vi "parametryKomor.vi"(3 "Akcja":T1, 4 "Wybór komory":T6, 5 "Wejœcie":T2={"Pinout"={"LEWO"=7, "PRAWO"=11, "GÓRA"=35, "Dӣ"=36, "CZUJNIK"=12}, "Parametry ruchu poziomego"={"Faza ruchu poziomego"=enum."Ruch", "Nr pozycji poziomej"=0, "Kolor czujnika"=FALSE, "Lista punków w poziomie"=[]}, "Parametry ruchy pionowego"={"Faza ruchu"=enum."Ruch", "Lista punktów w pionie"=[]}}) -> (2 "Wyjscie":T2={"Pinout"={"LEWO"=7, "PRAWO"=11, "GÓRA"=35, "Dӣ"=36, "CZUJNIK"=12}, "Parametry ruchu poziomego"={"Faza ruchu poziomego"=enum."Ruch", "Nr pozycji poziomej"=0, "Kolor czujnika"=FALSE, "Lista punków w poziomie"=[]}, "Parametry ruchy pionowego"={"Faza ruchu"=enum."Ruch", "Lista punktów w pionie"=[]}})   [LabVIEW 2014]
uses:
  parametryKomorVIs/WyborKomory.ctl
  parametryKomorVIs/Parametry_ramienia.ctl
  poziomyVIs/ParametryRuchuPoziomego.ctl
  Faza_ruchu.ctl
  pionowyVIs/ParametryRuchyPionowego.ctl
  AkcjaGFV.ctl
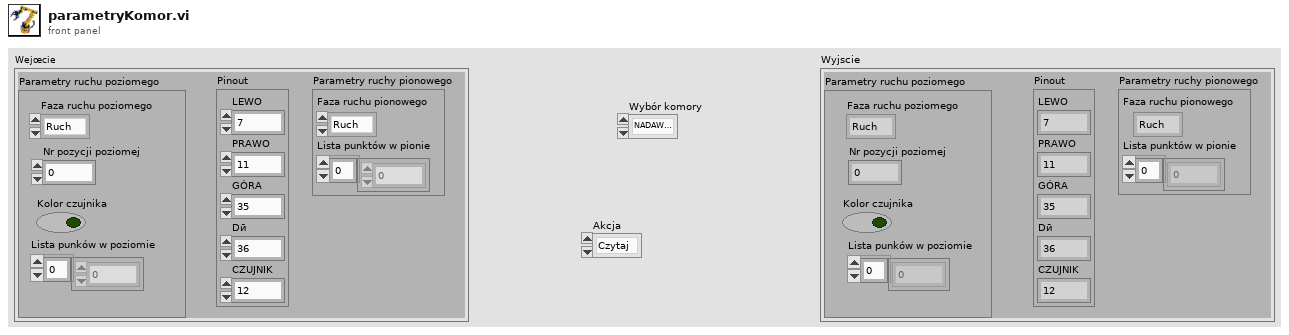
[diagram p1: front panel]
types:
  T1 = typedef "AkcjaGFV.ctl" = enum16{"Czytaj", "Zapisz", "Reset"}
  T2 = typedef "Parametry_ramienia.ctl" = cluster{"Pinout":cluster{"LEWO":u8, "PRAWO":u8, "GÓRA":u8, "Dӣ":u8, "CZUJNIK":u8}, "Parametry ruchu poziomego":T3, "Parametry ruchy pionowego":T5}
  T3 = typedef "ParametryRuchuPoziomego.ctl" = cluster{"Faza ruchu poziomego":T4, "Nr pozycji poziomej":i32, "Kolor czujnika":bool, "Lista punków w poziomie":i32[]}
  T4 = typedef "Faza_ruchu.ctl" = enum16{"Ruch", "Poczekaj", "Pomiar"}
  T5 = typedef "ParametryRuchyPionowego.ctl" = cluster{"Faza ruchu":T4, "Lista punktów w pionie":i32[]}
  T6 = typedef "WyborKomory.ctl" = enum16{"NADAWCZA", "ODBIORCZA"}
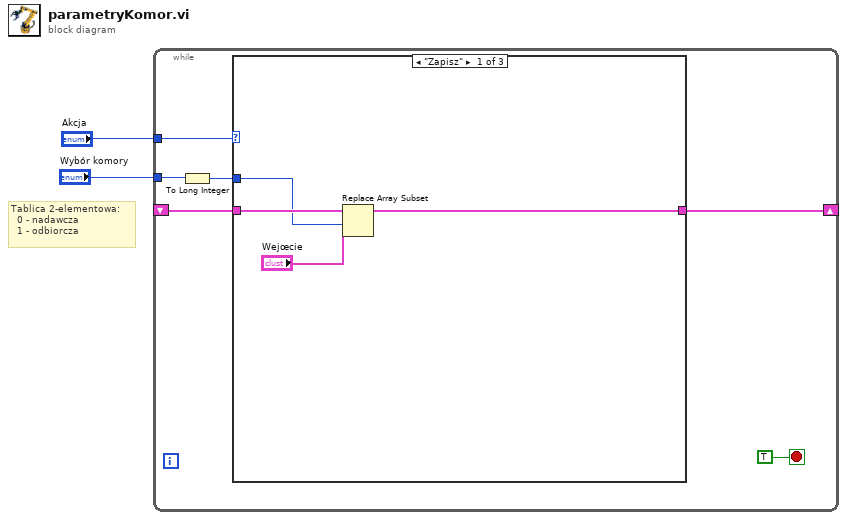
[diagram p0: block diagram]
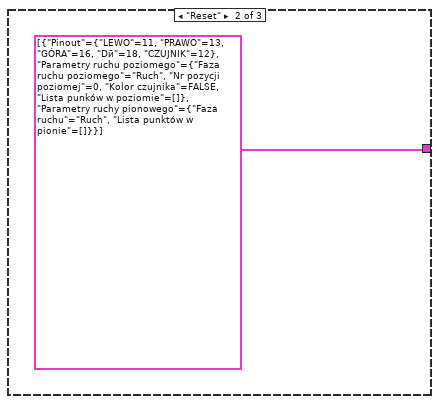
[diagram p2: hidden frame]
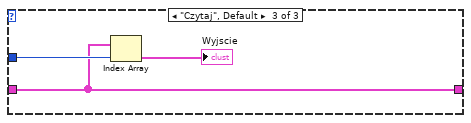
[diagram p3: hidden frame]
diagram:
  # "Tablica 2-elementowa: \n  0 - nadawcza\n  1 - odbiorcza"
  n1 = while {
    tunnel: "Wybór komory" -> [w4]
    shift-right: [w5] -> _
    shift-left: _ -> [w6]
    tunnel: "Akcja" -> [w7]
    stop <- TRUE stop-if-true
    n2 = To Long Integer(number=w4) -> (32bit integer=w3:i32)
    n3 = case shown="\"Zapisz\"" w7 {
      tunnel: w6 -> [w10 _ w15]
      tunnel: [w11 T2[] [{"Pinout"={"LEWO"=11, "PRAWO"=13, "GÓRA"=16, "Dӣ"=18, "CZUJNIK"=12}, "Parametry ruchu poziomego"={"Faza ruchu poziomego"=enum."Ruch", "Nr pozycji poziomej"=0, "Kolor czujnika"=FALSE, "Lista punków w poziomie"=[]}, "Parametry ruchy pionowego"={"Faza ruchu"=enum."Ruch", "Lista punktów w pionie"=[]}}] w15] -> w5
      tunnel: w3 -> [w9 _ w16]
      frame "Zapisz" {
        n4 = Replace Array Subset(array=w10, new element="Wejœcie", index=w9) -> (w11:T2[])
      }
      frame "Reset" {
      }
      frame "Czytaj", Default {
        n5 = Index Array(array=w15, index=w16) -> (element=→"Wyjscie":T2)
      }
    }
  }
